vi "Save_Source.vi"(8 "error in (no error)":errorcluster, 11 "Installer in":refnum<class "Installer.lvclass">) -> (0 "error out":errorcluster, 3 "Installer out":refnum<class "Installer.lvclass">)   [LabVIEW 2020, in "Installer.lvclass"]
uses:
  <vilib>/AppBuilder/IB_Classes/Installer/Installer.lvclass
  <vilib>/AppBuilder/IB_Classes/Installer/Installer.lvclass/Installer.ctl
  <vilib>/AppBuilder/IB_Classes/Source/IB_Source.lvclass
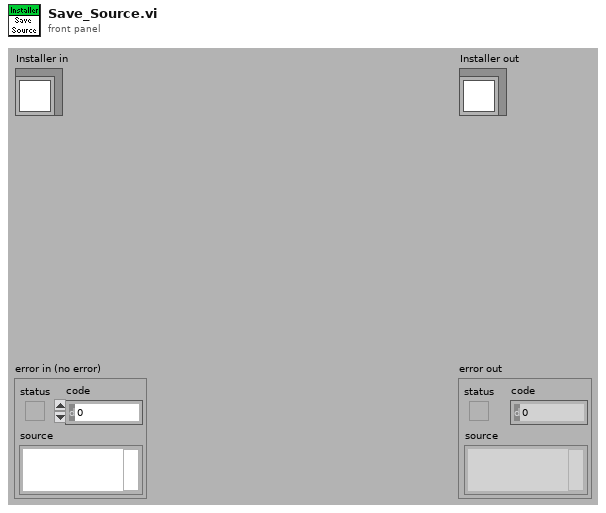
[diagram p1: front panel]
types:
  T1 = typedef "ItemRef.ctl" = u64
  T2 = typedef "IB_Source.ctl" = cluster{"name":string, "sourceTag":string, "destTag":string, "path":path, "eng_installPath":string, "UI_inBuild?":bool, "str ref?":bool}
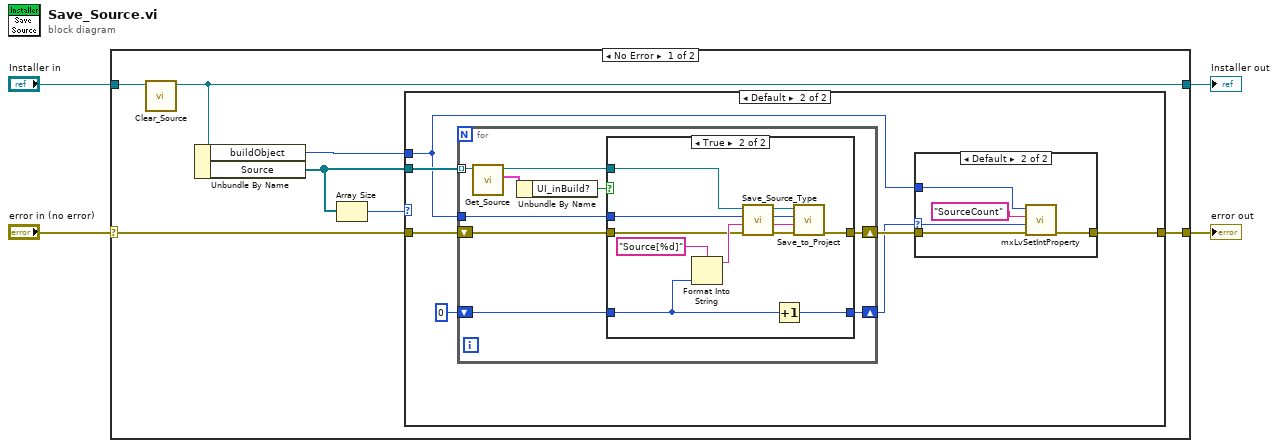
[diagram p0: block diagram]
diagram:
  n1 = case shown="No Error" "error in (no error)" {
    selector: "error in (no error)" -> [w5 w50]
    tunnel: [w6 w50] -> w3
    tunnel: [w8 w49] -> w1
    tunnel: "Installer in" -> [w9 w49]
    frame No Error {
      n2 = call-dynamic "Clear_Source.vi"("Installer in"=w9) -> ("Installer out"=w8:refnum<class "Installer.lvclass">)  [unwired: 9 in, 1 out]
      n3 = Unbundle By Name(w8) -> ("buildObject"=w10:T1, "Source"=w11:refnum<class "IB_Source.lvclass">[])
      n4 = Array Size(array=w11) -> (size(s)=w7:i32)
      n5 = case shown="Default" w7 {
        tunnel: w11 -> [_ w19]
        tunnel: w10 -> [_ w14]
        tunnel: [w12 w16] -> w6
        tunnel: w5 -> [w12 w18]
        frame 0 {
        }
        frame Default {
          n6 = for {
            tunnel: w19 -> [w31] mode=indexing
            tunnel: w14 -> [w34]
            shift-right: [w33] -> w17
            shift-left: w18 -> [w32]
            shift-right: [w26] -> w13
            shift-left: 0 -> [w27]
            n7 = call <vilib>:"Get_Source.vi"("IB_Source in"=w31) -> ("data"=w29:T2, "IB_Source out"=w30:refnum<class "IB_Source.lvclass">)  [unwired: 8 in, 1 out]
            n8 = Unbundle By Name(w29) -> ("UI_inBuild?"=w28:bool)
            n9 = case shown="True" w28 {
              tunnel: w34 -> [_ w45]
              tunnel: [w36 w41] -> w33
              tunnel: w32 -> [w36 w40]
              tunnel: w30 -> [_ w39]
              tunnel: w27 -> [w35 w37]
              tunnel: [w35 w38] -> w26
              frame False {
              }
              frame True {
                n10 = Format Into String(format string="Source[%d]", w37) -> (resulting string=w43:string)  [unwired: 2 in, 1 out]
                n11 = call-dynamic "Save_Source_Type.vi"("error in (no error)"=w40, "index in"=w43, "buildObject"=w45, "Class in"=w39) -> ("error out"=w42:errorcluster, "index out"=w46:string, "buildObject out"=w47:T1, "Class out"=w48:refnum<class "IB_Source.lvclass">)  [unwired: 4 in]
                n12 = Increment(x=w37) -> (x+1=w38:i32)
                n13 = call-dynamic "Save_to_Project.vi"("error in (no error)"=w42, "index in"=w46, "buildObject"=w47, "Class in"=w48) -> ("error out"=w41:errorcluster)  [unwired: 3 in, 4 out]
              }
            }
          }
          n14 = case shown="Default" w13 {
            selector: w13 -> [_ w21]
            tunnel: w17 -> [w20 w24]
            tunnel: [w20 w23] -> w16
            tunnel: w14 -> [_ w22]
            frame 0 {
            }
            frame Default {
              n15 = call <resource>:"mxLvSetIntProperty.vi"("error in"=w24, "Value (0)"=w21, "Tag"="SourceCount", "Item"=w22) -> ("error out"=w23:errorcluster)  [unwired: 6 in, 1 out]
            }
          }
        }
      }
    }
    frame Error {
    }
  }
  "error out" <- w3
  "Installer out" <- w1
